vi "Read Analog Input Values.vi"(8 "error in":errorcluster, 9 "Timeout / s":dbl=10.0 format="%0.2f", 10 "AI DAQmx Task":refnum<k21>, 11 "BNT_DAQmx-MCSV-AIAvg in":refnum<class "BNT_DAQmx-MCSV-AIAvg.lvclass">) -> (0 "error out":errorcluster, 1 "AI Data":dbl[](array[numeric]), 3 "BNT_DAQmx-MCSV-AIAvg out":refnum<class "BNT_DAQmx-MCSV-AIAvg.lvclass">)   [LabVIEW 2021, in "BNT_DAQmx.lvlib" / "BNT_DAQmx-MCSV-AIAvg.lvclass"]
doc: "Read analog input.\n\n<b>Default Implementation:</b> Analog Input\n\nThis dynamic dispatch VI can be overritten by derived classes to implement other analog input readings."
uses:
  BNT_DAQmx-MCSV-AIAvg.lvclass
  D:/Brand/LVP/Acc/VacuumHeating/Packages/CSPP_Core/Actors/CSPP_BaseActor/CSPP_BaseActor.lvclass
  BNT_DAQmx-MCSV-AIAvg.lvclass/BNT_DAQmx-MCSV-AIAvg.ctl
  CSPP_Core/Libraries/Base/Severity.ctl
  CSPP_Core/Actors/CSPP_BaseActor/CSPP_BaseActor.lvclass/CSPP_BaseActor.ctl
  <vilib>/DAQmx/read.llb/DAQmx Read (Analog 2D DBL NChan NSamp).vi
  <vilib>/Analysis/baseanly.llb/Mean (DBL).vi
  <vilib>/DAQmx/miscellaneous.llb/DAQmx Fill In Error Info.vi
  <vilib>/Analysis/NI_AALBase.lvlib
  CSPP_Core/Libraries/Utilities/CSPP_Utilities.lvlib
  CSPP_Core/Actors/CSPP_BaseActor/CSPP_BaseActor.lvclass
  CSPP_Core/Libraries/Base/CSPP_Base.lvlib
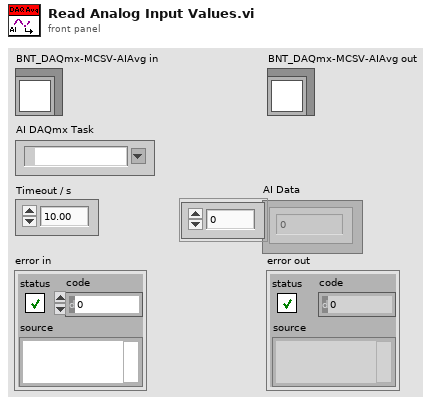
[diagram p1: front panel]
types:
  T1 = typedef "CSPP_Base.lvlib/Severity.ctl" = enum16{"emergency", "alert", "critical", "error", "warning", "notice", "info", "debug"}
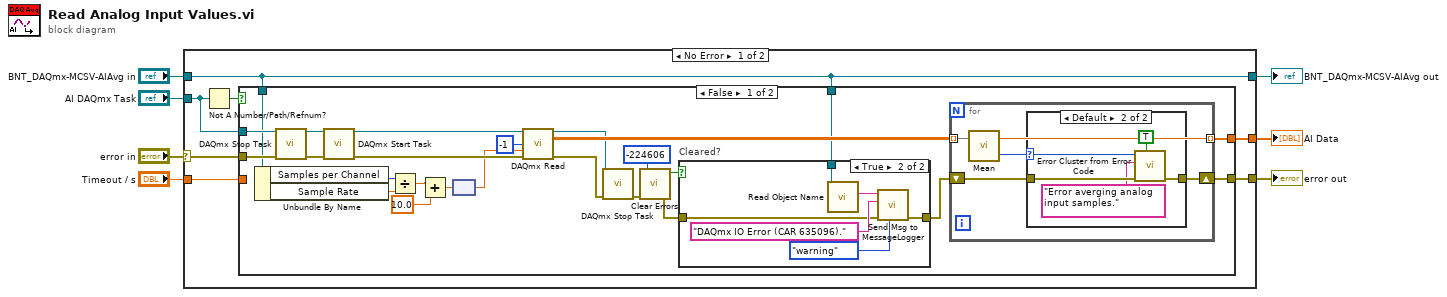
[diagram p0: block diagram]
diagram:
  n1 = case shown="No Error" "error in" {
    selector: "error in" -> [w13 w60]
    tunnel: [w12 w60] -> w2
    tunnel: [w8 w59] -> w4
    tunnel: "BNT_DAQmx-MCSV-AIAvg in" -> [w8 w59]
    tunnel: "Timeout / s" -> [w14 _]
    tunnel: [w11 _] -> w3
    tunnel: "AI DAQmx Task" -> [w9 _]
    frame No Error {
      n2 = Not A Number/Path/Refnum?(number/path/refnum=w9) -> (NaN/Path/Refnum?=w10:bool)
      n3 = case shown="False" w10 {
        tunnel: w14 -> [_ _]
        tunnel: w13 -> [w23 w58]
        tunnel: [w36 w58] -> w12
        tunnel: [w37 _] -> w11
        tunnel: w9 -> [w39 _]
        tunnel: w8 -> [w29 _]
        tunnel: w8 -> [w21 _]
        frame False {
          n4 = Unbundle By Name(w21) -> ("Samples per Channel"=w20:i32, "Sample Rate"=w19:dbl[unit])
          n5 = call <vilib>:"DAQmx Stop Task.vi"("task/channels in"=w39, "error in"=w23) -> ("task out"=w24:refnum<k21>, "error out"=w22:errorcluster)  [unwired: 12 in]
          n6 = call <vilib>:"DAQmx Start Task.vi"("task/channels in"=w24, "error in"=w22) -> ("task out"=w35:refnum<k21>, "error out"=w34:errorcluster)  [unwired: 12 in]
          n7 = Divide(x=w20, y=w19) -> (x/y=w16:dbl[unit])
          n8 = Add(x=w16, y=dbl[unit] 10.0) -> (x+y=w17:dbl[unit])
          n9 = node(w17) -> (w18:dbl)
          n10 = call-poly <vilib>:"DAQmx Read.vi"("task/channels in"=w35, "number of samples per channel"=-1, "timeout"=w18, "error in"=w34) -> ("task out"=w33:refnum<k21>, "data"=w38:dbl[][], "error out"=w32:errorcluster)  [unwired: 9 in]
          n11 = call <vilib>:"DAQmx Stop Task.vi"("task/channels in"=w33, "error in"=w32) -> ("error out"=w28:errorcluster)  [unwired: 12 in, 1 out]
          n12 = call <vilib>:"Clear Errors.vi"("error in (no error)"=w28, "specific error code to clear (0: all)"=-224606) -> ("error out"=w27:errorcluster, "specific error cleared?"=w25:bool)  [unwired: 4 in]
          n13 = case "Cleared?" shown="True" w25 {
            tunnel: w29 -> [_ w46]
            tunnel: w27 -> [w40 w43]
            tunnel: [w40 w42] -> w26
            frame False {
            }
            frame True {
              n14 = call "Read Object Name.vi"("CSPP_BaseActor in"=w46) -> ("Object Name"=w45:string)  [unwired: 8 in, 2 out]
              n15 = call "Send Msg to MessageLogger.vi"("Severity Code (info)"=Severity."warning", "Error In"=w43, "Message Content"="DAQmx IO Error (CAR 635096).", "Message Tag"=w45) -> ("Error Out"=w42:errorcluster)  [unwired: 7 in]
            }
          }
          n16 = for {
            tunnel: w38 -> [w51] mode=indexing
            tunnel: [w50] -> w37 mode=indexing
            shift-right: [w48] -> w36
            shift-left: w26 -> [w47]
            n17 = call-poly <vilib>:"Mean.vi"("X"=w51) -> ("mean"=w50:dbl, "error"=w49:i32)
            n18 = case shown="Default" w49 {
              selector: w49 -> [_ w57]
              tunnel: [w52 w56] -> w48
              tunnel: w47 -> [w52 w55]
              frame 0 {
              }
              frame Default {
                n19 = call "Error Cluster from Error Code.vi"("show call chain? (False)"=TRUE, "Error In"=w55, "Error Message (\"\")"="Error averging analog input samples." ("error message (\"\")"), "Error Code (0)"=w57) -> ("Error Out"=w56:errorcluster)  [unwired: 7 in]
              }
            }
          }
        }
        frame True {
        }
      }
    }
    frame Error {
    }
  }
  "error out" <- w2
  "BNT_DAQmx-MCSV-AIAvg out" <- w4
  "AI Data" <- w3
